vi "9601 Error Retrieving Base from Integer String--error.vi"(8 "error in":errorcluster, 11 "Integer String":string) -> (0 "error out":errorcluster)   [LabVIEW 2020, in "CANopen.lvlib"]
uses:
  CANopen.lvlib
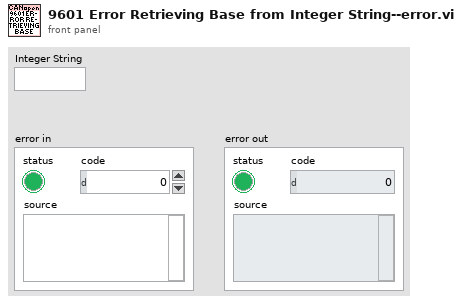
[diagram p1: front panel]
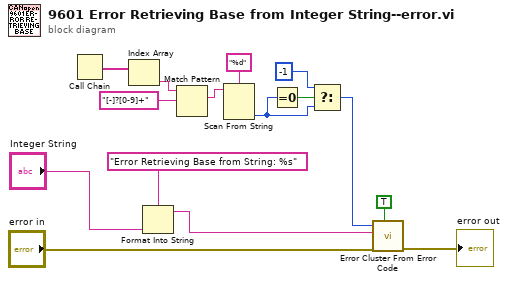
[diagram p0: block diagram]
diagram:
  n1 = Call Chain() -> (call chain=w9:string[])
  n2 = Index Array(array=w9) -> (element=w3:string)  [unwired: 1 in]
  n3 = Format Into String(format string="Error Retrieving Base from String: %s", "Integer String") -> (resulting string=w13:string)  [unwired: 2 in, 1 out]
  n4 = Match Pattern(string=w3, regular expression="[-]?[0-9]+") -> (match substring=w2:string)  [unwired: 1 in, 3 out]
  n5 = Scan From String(format string="%d", input string=w2) -> (output 1=w6:i32)  [unwired: 3 in, 3 out]
  n6 = Equal To 0?(x=w6) -> (x = 0?=w5:bool)
  n7 = Select(t=-1, s=w5, f=w6) -> (s? t:f=w8:i32)
  n8 = call <vilib>:"Error Cluster From Error Code.vi"("show call chain? (False)"=TRUE, "error in (no error)"="error in", "error message (\"\")"=w13, "error code (0)"=w8) -> ("error out"=→"error out":errorcluster)  [unwired: 5 in]
